vi "FIU Control - Channel.vi"() -> ()   [LabVIEW 2011]
doc: "Sample numeric display item."
uses:
  <vilib>/NI Veristand/Display Template Support/Display Template Support.llb/cluster_Screen Item Settings.ctl
  <vilib>/NI Veristand/Display Template Support/Display Template Support.llb/cluster_Graph Scale Settings.ctl
  <vilib>/NI Veristand/Display Template Support/Display Template Support.llb/cluster_Graph Plot Settings.ctl
  NationalInstruments.VeriStand.SystemStorage
  Channel Fault Selector.ctl
  <vilib>/NI Veristand/Display Template Support/Display Template Support.llb/enum_Display Template Handler Minimal To Widget Msg.ctl
  <vilib>/NI Veristand/Display Template Support/Display Template Support.llb/enum_Display Template Handler Minimal To Workspace.ctl
  <vilib>/NI Veristand/Display Template Support/Display Template Support.llb/sub_Display Template Handler Custom.vi
  <vilib>/NI Veristand/Execution/Workspace/NI VeriStand - Get Single Channel Value.vi
  <vilib>/NI Veristand/Execution/Workspace/NI VeriStand - Set Single Channel Value.vi
  <vilib>/NI Veristand/Execution/Workspace/NI_VS Workspace ExecutionAPI.lvlib
panel:
  in  "Enum":T1
  in  "NIVS.System Definition Root":refnum<k24>
  in  "NIVS.Gateway IP Address":string
  out "Label":string="Numeric"
  in  "Item.Data":T2
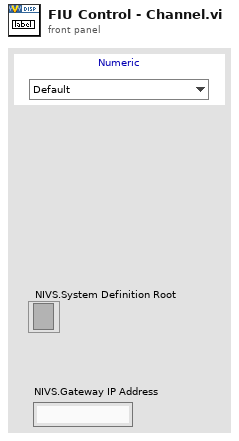
[diagram p1: front panel]
types:
  T1 = typedef "Channel Fault Selector.ctl" = enum16{"Default", "DUT Pass Through", "DUT Open", "DUT Pass Through and FB A", "DUT Pass Through and FB B", "DUT FB A", "DUT FB B"}
  T2 = typedef "cluster_Screen Item Settings.ctl" = cluster{"Template VI":string, "Position X":i32, "Position Y":i32, "Custom":string, "Show Title Bar":bool, "ID":i32, "Always On Top":bool, "Allow Resize":bool, "Allow Minimize":bool, "Allow Close":bool, "Size to Screen":bool, "Screen.ID":i32, "State":enum16{"Normal", "New"}, "Title":string, "Window Bounds":cluster{"[0]":i16, "[1]":i16, "[2]":i16, "[3]":i16}, "Channel Ref":u64, "Unit":string, "Default Units?":bool, "Flash Limit?":bool, "Color 1":u32, "Color 2":u32, "Color 3":u32, "Color 4":u32, "Bck Color":u32, "Fore Color":u32, "Limit 1":dbl, "Limit 2":dbl, "Limit 3":dbl, "Limit 4":dbl, "Limit Mode 1":i32, "Limit Mode 2":i32, "Limit Mode 3":i32, "Limit Mode 4":i32, "Scale Precision":i32, "Scale Min":dbl, "Scale Max":dbl, "Format":i32, "Precision":i32, "Background Type":i32, "IDs":i32[], "Units":string[], "Labels":string[], "Scale Factor":dbl, "Scale Offset":dbl, "YScale Index":u32[], "XScale":T3, "YScales":T3[], "Plots":T4[], "Update Period":dbl, "History Length":dbl, "My.Ref":refnum<vi>, "Is Control?":bool, "Channel Paths":string[], "Custom Data":variant}
  T3 = typedef "cluster_Graph Scale Settings.ctl" = cluster{"Format":u8, "Precision":u8, "Fit":u8, "Label":string, "Use Default Label":bool, "Label Visible":bool, "Min":dbl, "Max":dbl}
  T4 = typedef "cluster_Graph Plot Settings.ctl" = cluster{"Bar Style":u8, "Fill To":i16, "Fill/PtColor":u32, "Line Style":u8, "Line Width":u8, "Color":u32, "Interp":u8, "Point Style":u8}
  T5 = typedef "enum_Display Template Handler Minimal To Workspace.ctl" = cluster{"Operation":enum16{"SetCustomData", "DeleteItem"}, "Data":variant}
  T6 = typedef "enum_Display Template Handler Minimal To Widget Msg.ctl" = enum16{"Stop", "LaunchConfigDialog"}
  T7 = typedef "NI_VS Workspace ExecutionAPI.lvlib/WorkspaceAPI.ctl" = refnum<k24>
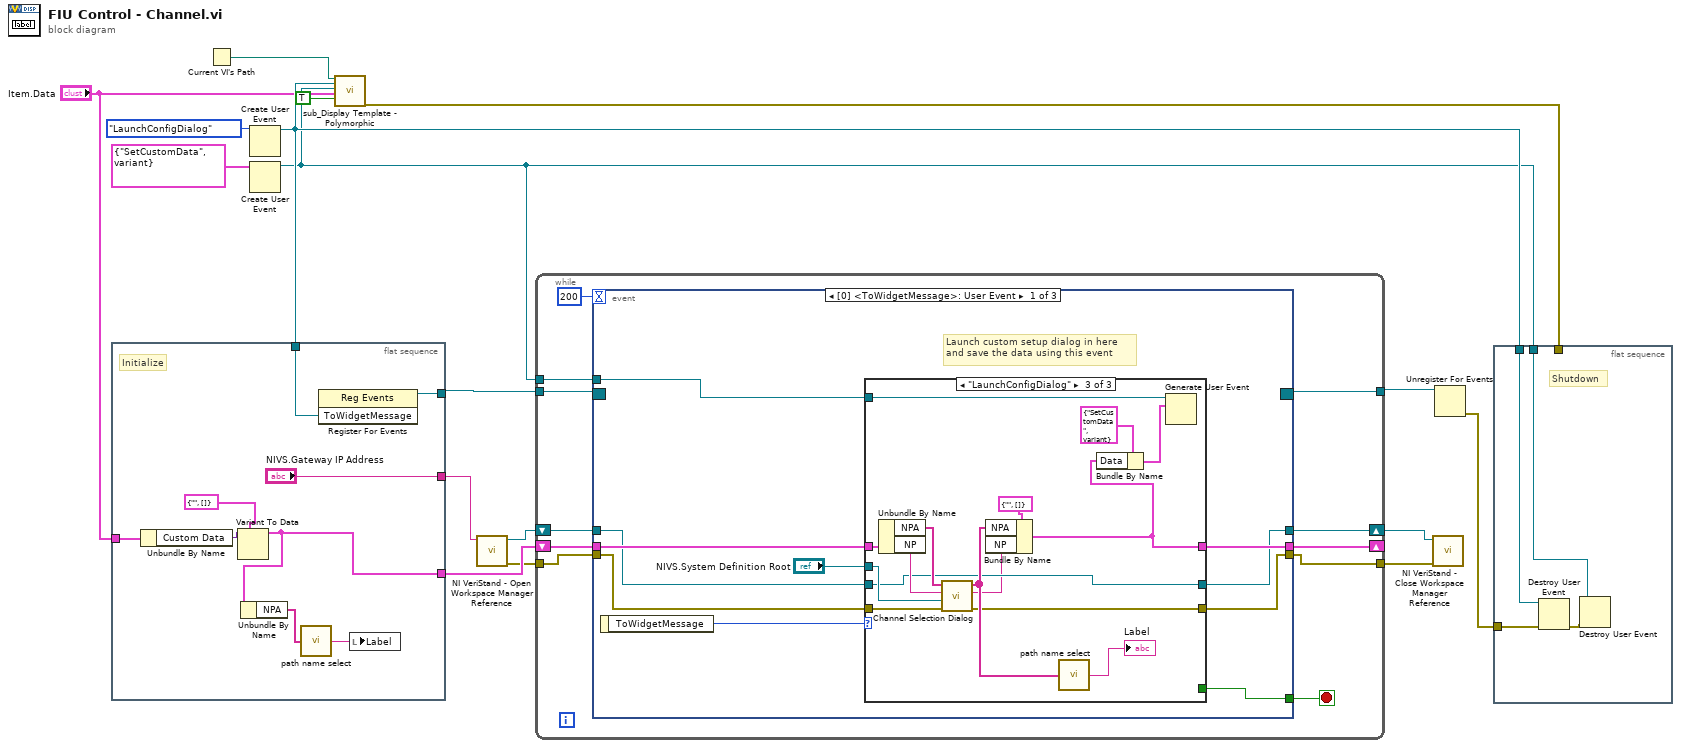
[diagram p0: block diagram]
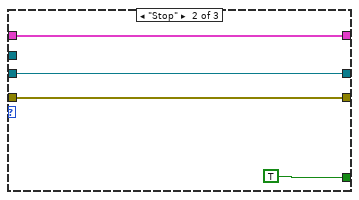
[diagram p3: hidden frame]
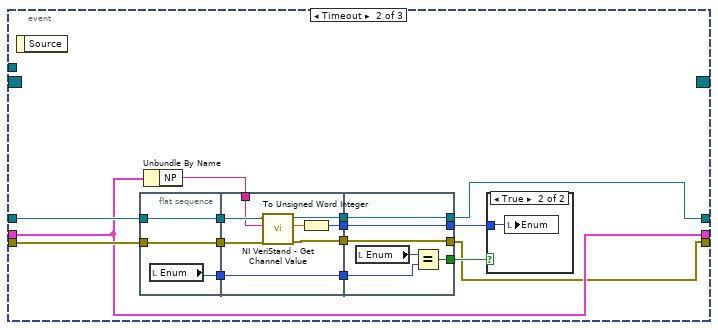
[diagram p4: hidden frame]
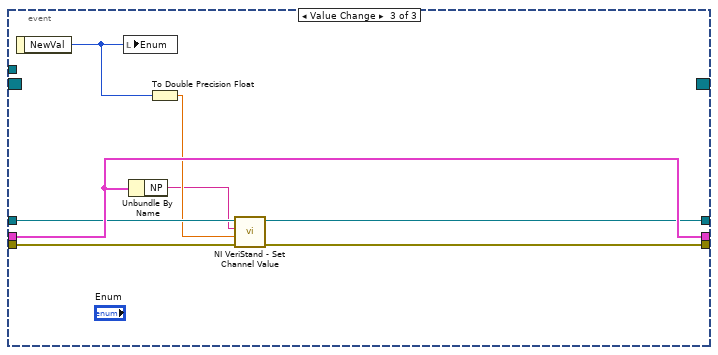
[diagram p6: hidden frame]
diagram:
  n1 = flat-sequence {
    tunnel: [w26] -> w15
    tunnel: w12 -> [w25]
    tunnel: "Item.Data" -> [w24]
    tunnel: [w20] -> w6
    tunnel: ["NIVS.Gateway IP Address"] -> w2
    frame #0 {
      # "Initialize"
      n2 = Unbundle By Name(w24) -> ("Custom Data"=w23:variant)
      n3 = Variant To Data(type=cluster{"NP":string, "NPA":string[]} {"NP"="", "NPA"=[]}, Variant=w23) -> (data=w20:cluster{"NP":string, "NPA":string[]})  [unwired: 1 in, 1 out]
      n4 = Unbundle By Name(w20) -> ("NPA"=w19:string[])
      n5 = call "path name select.vi"("NodePathArray"=w19) -> ("Label"=w18:string)
      n6 = register-events(w25) -> (reference out=w26:refnum<event-registration>)  [unwired: 2 in, 1 out]
      n7 = local write "Label"(w18) -> ()
    }
  }
  n8 = Current VI's Path() -> (path=w10:path)
  n9 = Create User Event(user event datatype=enum_Display_Template_Handler_Minimal_To_Widget_Msg."LaunchConfigDialog" ("ToWidgetMessage")) -> (user event=w12:refnum<user-event>)  [unwired: 1 in, 1 out]
  n10 = Create User Event(user event datatype=T5 {"Operation"=enum."SetCustomData", "Data"=variant} ("Data")) -> (user event=w8:refnum<user-event>)  [unwired: 1 in, 1 out]
  n11 = call-poly <vilib>:"sub_Display Template - Polymorphic.vi"("Parent.Path"=w10, "ToWidgetEvent"=w12, "ToWorkspace"=w8, "Item.Data"="Item.Data", "Resizable"=TRUE) -> ("error out"=w17:errorcluster)  [unwired: 1 in, 13 out]
  n12 = call <vilib>:"NI VeriStand - Open Workspace Manager Reference.vi"("Gateway IP Address (\"\": localhost)"=w2) -> ("error out"=w1:errorcluster, "WorkspaceManager"=w5:T7)  [unwired: 9 in]
  n13 = while {
    tunnel: w15 -> [w37]
    tunnel: [w35] -> w14
    tunnel: w8 -> [w34]
    shift-right: [w28] -> _
    shift-left: w6 -> [w33]
    shift-right: [w29] -> w4
    shift-left: w5 -> [w31]
    tunnel: w1 -> [w30]
    tunnel: [w27] -> w3
    stop <- w36 stop-if-true
    n14 = event shown="[0] <ToWidgetMessage>: User Event" {
      selector: w37 -> [_ _ _]
      dyn-events: [_ _ _] -> w35
      timeout: 200 -> [_ _ _]
      tunnel: [w46 _ _] -> w36
      tunnel: w34 -> [w45 _ _]
      tunnel: [w44 w81 w110] -> w28
      tunnel: w33 -> [w43 w81 w110]
      tunnel: w31 -> [w42 w83 w108]
      tunnel: w30 -> [w41 w84 w109]
      tunnel: [w40 w82 w106] -> w29
      tunnel: [w39 w70 w105] -> w27
      event User Event {
        # "Launch custom setup dialog in here\nand save the data using this event"
        n15 = event-data() -> ("ToWidgetMessage"=w47:T6)  [unwired: 1 out]
        n16 = case shown="\"LaunchConfigDialog\"" w47 {
          tunnel: [_ TRUE _] -> w46
          tunnel: w45 -> [_ _ w69]
          tunnel: [w50 w53 w61] -> w44
          tunnel: w43 -> [w50 w53 w64]
          tunnel: w42 -> [w49 w52 w57]
          tunnel: w41 -> [w48 w51 w66]
          tunnel: [w49 w52 w57] -> w40
          tunnel: [w48 w51 w58] -> w39
          tunnel: "NIVS.System Definition Root" -> [_ _ w65]
          frame Default {
          }
          frame "Stop" {
          }
          frame "LaunchConfigDialog" {
            n17 = Unbundle By Name(w64) -> ("NPA"=w62:string[], "NP"=w63:string)
            n18 = call "Channel Selection Dialog.vi"("error in (no error)"=w66, "NIVS.System Definition Root"=w65, "NodePath"=w63, "NodePathArray"=w62) -> ("error out"=w58:errorcluster, "Selected NodePath"=w55:string, "Selected NodePathArray"=w59:string[])  [unwired: 5 in]
            n19 = Bundle By Name(cluster=cluster{"NP":string, "NPA":string[]} {"NP"="", "NPA"=[]}, "NPA"=w59, "NP"=w55) -> (w61:cluster{"NP":string, "NPA":string[]})
            n20 = call "path name select.vi"("NodePathArray"=w59) -> ("Label"=→"Label":string)
            n21 = Bundle By Name(cluster=T5 {"Operation"=enum."SetCustomData", "Data"=variant} ("event data"), "Data"=w61) -> (w67:T5)
            n22 = Generate User Event(user event=w69, event data cluster=w67) -> ()  [unwired: 1 in, 2 out]
          }
        }
      }
      event Timeout {
        n23 = event-data() -> ()  [unwired: 2 out]
        n24 = flat-sequence {
          tunnel: w83 -> [w86]
          tunnel: w84 -> [w87]
          tunnel: [w87] -> w79
          tunnel: [w86] -> w78
          tunnel: [w85] -> w73
          tunnel: w80 -> [w92]
          tunnel: w79 -> [w95]
          tunnel: w78 -> [w94]
          tunnel: [w93] -> w76
          tunnel: [w90] -> w75
          tunnel: w73 -> [w89]
          tunnel: [w89] -> w72
          tunnel: [w88] -> w71
          tunnel: [w100] -> w77
          tunnel: [w101] -> w82
          tunnel: w76 -> [w101]
          tunnel: w75 -> [w100]
          tunnel: [w99] -> w74
          tunnel: w72 -> [w97]
          tunnel: [w96] -> w70
          tunnel: w71 -> [w96]
          frame #0 {
            n25 = local read "Enum"() -> (w85:T1)
          }
          frame #1 {
            n26 = call-poly <vilib>:"NI VeriStand - Get Channel Value.vi"("error in (no error)"=w95, "Channel"=w92, "WorkspaceManager in"=w94) -> ("error out"=w88:errorcluster, "Value"=w91:dbl, "WorkspaceManager out"=w93:T7)  [unwired: 6 in]
            n27 = To Unsigned Word Integer(number=w91) -> (unsigned 16bit integer=w90:u16)
          }
          frame #2 {
            n28 = local read "Enum"() -> (w98:T1)
            n29 = Equal?(x=w98, y=w97) -> (x = y?=w99:bool)
          }
        }
        n30 = Unbundle By Name(w81) -> ("NP"=w80:string)
        n31 = case shown="True" w74 {
          tunnel: w77 -> [_ w102]
          frame False {
          }
          frame True {
            n32 = local write "Enum"(w102) -> ()
          }
        }
      }
      event Value Change {
        n33 = event-data() -> ("NewVal"=w103:T1)  [unwired: 1 out]
        n34 = local write "Enum"(w103) -> ()
        n35 = Unbundle By Name(w110) -> ("NP"=w104:string)
        n36 = To Double Precision Float(number=w103) -> (double precision float=w107:dbl)
        n37 = call-poly <vilib>:"NI VeriStand - Set Channel Value.vi"("error in (no error)"=w109, "Value"=w107, "Channel"=w104, "WorkspaceManager in"=w108) -> ("error out"=w105:errorcluster, "WorkspaceManager out"=w106:T7)  [unwired: 6 in]
      }
    }
  }
  n38 = call <vilib>:"NI VeriStand - Close Workspace Manager Reference.vi"("error in (no error)"=w3, "WorkspaceManager"=w4) -> ()  [unwired: 9 in, 1 out]
  n39 = Unregister For Events(event registration refnum=w14) -> (error out=w13:errorcluster)  [unwired: 1 in]
  n40 = flat-sequence {
    tunnel: w17 -> [_]
    tunnel: w13 -> [w113]
    tunnel: w12 -> [w114]
    tunnel: w8 -> [w111]
    frame #0 {
      # "Shutdown"
      n41 = Destroy User Event(user event=w114, error in=w113) -> (error out=w112:errorcluster)
      n42 = Destroy User Event(user event=w111, error in=w112) -> ()  [unwired: 1 out]
    }
  }
